vi "AssetInterface_Initalize Assets.vi"(8 "error in (no error)":errorcluster, 11 "Grid in":refnum<class "Grid.lvclass">) -> (0 "error out":errorcluster, 2 "TagDescriptions":refnum<class "tag descriptor.lvclass">[](array[class]), 3 "Grid out":refnum<class "Grid.lvclass">)   [LabVIEW 2015, in "Grid.lvclass"]
uses:
  Grid.lvclass
  <vilib>/NI/Tag Bus/tag/tag descriptor.lvclass
  TagBus/TagBus.lvclass
panel:
  out "Grid_Status":cluster{"kW":dbl}
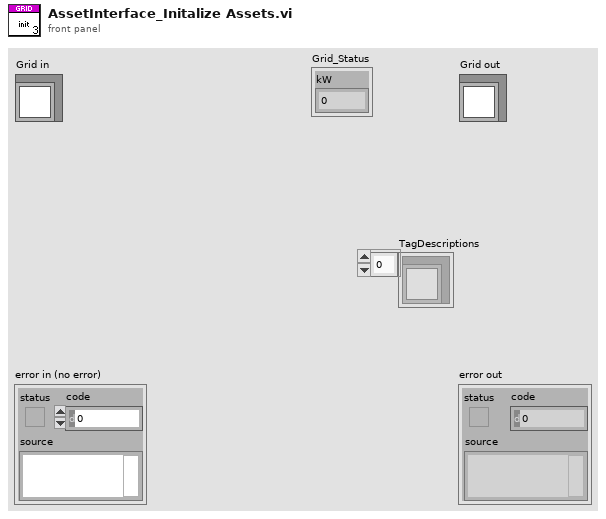
[diagram p1: front panel]
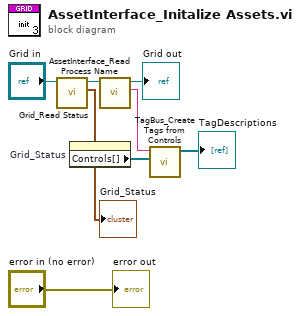
[diagram p0: block diagram]
diagram:
  n1 = call-dynamic "Grid_Read Status.vi"("Grid in"="Grid in") -> ("Grid_Status"=→"Grid_Status":cluster{"kW":dbl}, "Grid out"=w5:refnum<class "Grid.lvclass">)  [unwired: 9 in]
  n2 = property on="Grid_Status" class="Clust (strict)"() -> ("Controls[]"=w3:refnum<vi>[])  [unwired: 2 in, 2 out]
  n3 = call-dynamic "AssetInterface_Read Process Name.vi"("Grid in"=w5) -> ("Process Name"=w2:string, "Grid out"=→"Grid out":refnum<class "Grid.lvclass">)  [unwired: 9 in]
  n4 = call "TagBus_Create Tags from Controls.vi"("Array"=w3, "Process Name"=w2) -> ("TagDescriptions"=→"TagDescriptions":refnum<class "tag descriptor.lvclass">[])  [unwired: 9 in]
  "error out" <- "error in (no error)"
